vi "niFPGA Square Wave Generator.vi"(0 "frequency (periods/tick)":fxp<+,32,0>=0.00390625, 1 "reset":bool, 5 "phase offset (periods)":fxp<+,32,0>, 7 "duty cycle (periods)":fxp<+,32,0>=0.5, 12 "amplitude":i16=32767, 13 "offset":i16) -> (4 "square wave out":i16)   [LabVIEW 2017]
doc: "Generates a point-by-point square wave using direct digital synthesis (DDS). The synthesis runs continuously using the block diagram clock rate to produce a real-time frequency. The block diagram clock rate is the top-level clock rate, unless the Square Wave Generator Express VI is inside a single-cycle Timed Loop configured with a different clock rate."
uses:
  <vilib>/Platform/TimedLoop/XDataNode/timing_clust.ctl
  <vilib>/Platform/TimedLoop/XDataNode/nitl_modes.ctl
  <vilib>/Platform/TimedLoop/XDataNode/wakeup.ctl
  <vilib>/Platform/TimedLoop/XDataNode/XDataNode.xnode
  <vilib>/Platform/TimedLoop/XDataNode/XDNodeRunTimeDep.lvlib
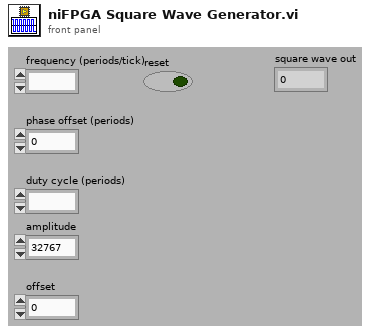
[diagram p1: front panel]
types:
  T1 = typedef "XDNodeRunTimeDep.lvlib/timing_clust.ctl" = cluster{"Expected End [f-1]":u64, "Actual End [f-1]":u64, "Finished Late? [f-1]":bool, "Expected End [i-1]":u64, "Actual End [i-1]":u64, "Finished Late? [i-1]":bool, "Expected Start [i]":u64, "Actual Start [i]":u64, "Expected Start [f]":u64, "Actual Start [f]":u64, "Source Name":string, "Structure Name":string, "Period":i64, "Deadline":i64, "Offset":i64, "Start":i64, "Priority":i32, "Timeout":i32, "Mode":T2, "Wakeup Reason":T3, "Error":errorcluster, "Source Type":string, "Secondary Source Type":string, "Global End Time":u64, "Global Start Time":u64, "Frame Duration":u64, "Iteration Duration":u64, "Assigned CPU":i32, "I/O Scan Engine Mode":u32}
  T2 = typedef "XDNodeRunTimeDep.lvlib/nitl_modes.ctl" = enum32{"No Change", "Process missed periods, maintain original phase", "Discard missed periods, maintain original phase", "Process missed periods, ignore original phase", "Discard missed periods, ignore original phase"}
  T3 = typedef "XDNodeRunTimeDep.lvlib/wakeup.ctl" = enum32{"Normal", "Aborted", "Asynchronous wakeup", "Timing source error", "Timed loop error", "Timeout"}
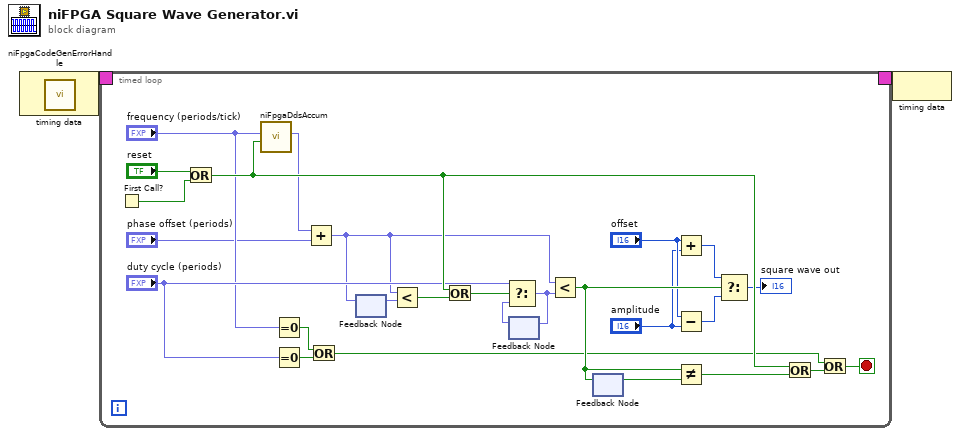
[diagram p0: block diagram]
diagram:
  n1 = node-c288() -> (w2:T1)  [unwired: 1 out]
  n2 = call <vilib>:"niFpgaCodeGenErrorHandle.vi"() -> ()  [unwired: 1 out]
  n3 = timed-loop "Timed Loop" {
    timing: w2 -> [_]
    timing-out: [_] -> w1
    stop <- w17 stop-if-true
    n4 = First Call?() -> (First Call?: T/F=w28:bool)
    n5 = Or(x="reset", y=w28) -> (x .or. y?=w27:bool)
    n6 = call <vilib>:"niFpgaDdsAccum.vi"("init"=w27, "frequency_scaled"="frequency (periods/tick)") -> ("current_accum_state"=w6:fxp<+,32,0>)  [unwired: 8 out]
    n7 = Equal To 0?(x="frequency (periods/tick)") -> (x = 0?=w23:bool)
    n8 = Equal To 0?(x="duty cycle (periods)") -> (x = 0?=w22:bool)
    n9 = Add(x=w6, y="phase offset (periods)") -> (x+y=w4:fxp<+,32,0>)
    n10 = Or(x=w23, y=w22) -> (x .or. y?=w21:bool)
    n11 = feedback-in #1(w4) -> ()
    n12 = feedback #1() -> (w7:fxp<+,32,0>)  [unwired: 1 out]
    n13 = Less?(x=w4, y=w7) -> (x < y?=w3:bool)
    n14 = Or(x=w27, y=w3) -> (x .or. y?=w14:bool)
    n15 = feedback #2() -> (w16:fxp<+,32,0>)  [unwired: 1 out]
    n16 = Select(t="duty cycle (periods)", s=w14, f=w16) -> (s? t:f=w15:fxp<+,32,0>)
    n17 = feedback-in #2(w15) -> ()
    n18 = Less?(x=w4, y=w15) -> (x < y?=w26:bool)
    n19 = feedback-in #3(w26) -> ()
    n20 = feedback #3() -> (w25:bool)  [unwired: 1 out]
    n21 = Add(x="offset", y="amplitude") -> (x+y=w19:i16)
    n22 = Subtract(x="offset", y="amplitude") -> (x-y=w18:i16)
    n23 = Not Equal?(x=w26, y=w25) -> (x != y?=w24:bool)
    n24 = Select(t=w19, s=w26, f=w18) -> (s? t:f=→"square wave out":i16)
    n25 = Or(x=w27, y=w24) -> (x .or. y?=w20:bool)
    n26 = Or(x=w21, y=w20) -> (x .or. y?=w17:bool)
  }
  n27 = node-c288(w1) -> ()
